vi "Capture ADC.vi"() -> ()   [LabVIEW 2023]
uses:
  <instrlib>/tio-labview/TIO Library/TIO Stream Open.vi
  <instrlib>/tio-labview/TIO Library/TIO RPC Send REQuest.vi
  <instrlib>/tio-labview/TIO Library/TIO RPC Parse Reply.vi
  <instrlib>/tio-labview/TIO Library/TIO RPC Parse Reply Error.vi
  <instrlib>/tio-labview/TIO Library/TIO Data Stream Parse timebase Info.vi
  <instrlib>/tio-labview/TIO Library/TIO Data Stream Parse pstream Info.vi
  <instrlib>/tio-labview/TIO Library/TIO Data Stream Parse dstream Info.vi
  <vilib>/Utility/High Resolution Relative Seconds.vi
  <vilib>/Utility/error.llb/Clear Errors.vi
  <instrlib>/tio-labview/Labview Signal Processing/Log Binning.vi
  <instrlib>/tio-labview/TIO Library/TIO Serial Port Name Search.vi
  <instrlib>/tio-labview/TIO Library/TIO Stream Write.vi
  <instrlib>/tio-labview/TIO Library/TIO RPC Form Request.vi
  <instrlib>/tio-labview/Labview Signal Processing/Log Range.vi
  <instrlib>/tio-labview/TIO Library/TIO SLIP Serial Write.vi
  <instrlib>/tio-labview/TIO Library/TIO Form Packet.vi
  <instrlib>/tio-labview/TIO Library/TIO SLIP Encode.vi
  <instrlib>/tio-labview/TIO Library/TIO Serial Checksum CRC32.vi
  <vilib>/Utility/tcp.llb/UDP Multicast Open.vi
  <vilib>/Utility/tcp.llb/UDP Multicast Read-Write Open.vi
  <instrlib>/tio-labview/TIO Library/TIO Serial Port Discovery.vi
  <vilib>/Instr/_visa.llb/VISA Configure Serial Port (Instr).vi
  <instrlib>/tio-labview/TIO Library/TIO RPC Blocking.vi
  <instrlib>/tio-labview/TIO Library/TIO Stream Read Non-blocking.vi
  <instrlib>/tio-labview/TIO Library/TIO RPC Send Heartbeat.vi
  <vilib>/Analysis/6fits.llb/General Polynomial Fit.vi
  <vilib>/measure/maspectr.llb/FFT Power Spectrum and PSD.vi
  <vilib>/measure/maspectr.llb/FFT Power Spectrum and PSD for 1 Chan.vi
panel:
  in  "Samples":u32
  in  "Auto Trigger":bool
  in  "Trigger":bool
  in  "Quit":bool
  out "ID":string
  in  "URL":refnum<visa-resource-name>="tcp://localhost"
  out "Waveform Graph":cluster{dbl, dbl, dbl[][]}(graph)
  in  "Bin":bool=TRUE
  out "XY Graph":T1(graph)=[{"Frequencies Binned"=[0.14367816091954022, 0.28735632183908044, 0.43103448275862066, 0.5747126436781609, 0.7183908045977011, 0.8620689655172413, 1.0057471264367814, 1.1494252873563218, 1.293103448275862, 1.4367816091954024, 1.5804597701149428, 1.724137931034483, 1.8678160919540234, 2.0114942528735638, 2.155172413793104, 2.2988505747126444, 2.4425287356321848, 2.586206896551725, 2.7298850574712654, 2.8735632183908058, 3.017241379310346, 3.1609195402298864, 3.3045977011494267, 3.448275862068967, 3.5919540229885074, 3.7356321839080477, 3.879310344827588, 4.022988505747128, 4.166666666666669, 4.310344827586209, 4.454022988505749, 4.59770114942529, 4.8132183908046, 5.028735632183911, 5.172413793103451, 5.316091954022991, 5.531609195402302, 5.747126436781612, 5.962643678160923, 6.178160919540233, 6.393678160919544, 6.6810344827586245, 6.896551724137935, 7.1120689655172455, 7.399425287356326, 7.686781609195407, 7.9741379310344875, 8.261494252873568, 8.548850574712649, 8.908045977011499, 9.267241379310349, 9.55459770114943, 9.91379310344828, 10.344827586206902, 10.704022988505752, 11.063218390804602, 11.494252873563227, 11.925287356321846, 12.356321839080467, 12.787356321839086, 13.290229885057478, 13.793103448275872, 14.295977011494262, 14.870689655172423, 15.445402298850585, 16.020114942528743, 16.5948275862069, 17.169540229885055, 17.816091954022976, 18.462643678160898, 19.10919540229882, 19.827586206896516, 20.54597701149421, 21.336206896551673, 22.126436781609133, 22.916666666666597, 23.778735632183825, 24.64080459770106, 25.57471264367806, 26.580459770114828, 27.586206896551598, 28.591954022988368, 29.597701149425138, 30.67528735632168, 31.824712643677987, 33.045977011494095, 34.26724137931019, 35.488505747126304, 36.85344827586195, 38.2183908045976, 39.58333333333324, 41.091954022988446, 42.600574712643635, 44.1810344827586, 45.83333333333334, 47.48563218390807, 49.28160919540235, 51.14942528735639, 53.017241379310434, 54.956896551724256, 56.96839080459785, 59.051724137931224, 61.27873563218412, 63.5775862068968, 65.94827586206915, 68.39080459770125, 70.9051724137931, 73.56321839080448, 76.29310344827564, 79.09482758620658, 82.04022988505704, 85.05747126436728, 88.14655172413728, 91.45114942528659, 94.89942528735543, 98.34770114942428, 101.93965517241267, 105.74712643678036, 109.69827586206759, 113.79310344827434, 117.95977011494085, 122.27011494252692, 126.86781609195204, 131.6091954022967, 136.42241379310113, 141.45114942528483, 146.69540229884782, 152.15517241379015, 157.8304597701118, 163.64942528735295, 169.6839080459734, 176.00574712643294, 182.5431034482718, 189.29597701148995, 196.2643678160874], "Spectrum Binned"=[nan, nan, nan, nan, nan, nan, nan, nan, nan, nan, nan, nan, nan, nan, nan, nan, nan, nan, nan, nan, nan, nan, nan, nan, nan, nan, nan, nan, nan, nan, nan, nan, nan, nan, nan, nan, nan, nan, nan, nan, nan, nan, nan, nan, nan, nan, nan, nan, nan, nan, nan, nan, nan, nan, nan, nan, nan, nan, nan, nan, nan, nan, nan, nan, nan, nan, nan, nan, nan, nan, nan, nan, nan, nan, nan, nan, nan, nan, nan, nan, nan, nan, nan, nan, nan, nan, nan, nan, nan, nan, nan, nan, nan, nan, nan, nan, nan, nan, nan, nan, nan, nan, nan, nan, nan, nan, nan, nan, nan, nan, nan, nan, nan, nan, nan, nan, nan, nan, nan, nan, nan, nan, nan, nan, nan, nan, nan, nan, nan, nan, nan, nan, nan, nan, nan]}, {"Frequencies Binned"=[0.14367816091954022, 0.28735632183908044, 0.43103448275862066, 0.5747126436781609, 0.7183908045977011, 0.8620689655172413, 1.0057471264367814, 1.1494252873563218, 1.293103448275862, 1.4367816091954024, 1.5804597701149428, 1.724137931034483, 1.8678160919540234, 2.0114942528735638, 2.155172413793104, 2.2988505747126444, 2.4425287356321848, 2.586206896551725, 2.7298850574712654, 2.8735632183908058, 3.017241379310346, 3.1609195402298864, 3.3045977011494267, 3.448275862068967, 3.5919540229885074, 3.7356321839080477, 3.879310344827588, 4.022988505747128, 4.166666666666669, 4.310344827586209, 4.454022988505749, 4.59770114942529, 4.8132183908046, 5.028735632183911, 5.172413793103451, 5.316091954022991, 5.531609195402302, 5.747126436781612, 5.962643678160923, 6.178160919540233, 6.393678160919544, 6.6810344827586245, 6.896551724137935, 7.1120689655172455, 7.399425287356326, 7.686781609195407, 7.9741379310344875, 8.261494252873568, 8.548850574712649, 8.908045977011499, 9.267241379310349, 9.55459770114943, 9.91379310344828, 10.344827586206902, 10.704022988505752, 11.063218390804602, 11.494252873563227, 11.925287356321846, 12.356321839080467, 12.787356321839086, 13.290229885057478, 13.793103448275872, 14.295977011494262, 14.870689655172423, 15.445402298850585, 16.020114942528743, 16.5948275862069, 17.169540229885055, 17.816091954022976, 18.462643678160898, 19.10919540229882, 19.827586206896516, 20.54597701149421, 21.336206896551673, 22.126436781609133, 22.916666666666597, 23.778735632183825, 24.64080459770106, 25.57471264367806, 26.580459770114828, 27.586206896551598, 28.591954022988368, 29.597701149425138, 30.67528735632168, 31.824712643677987, 33.045977011494095, 34.26724137931019, 35.488505747126304, 36.85344827586195, 38.2183908045976, 39.58333333333324, 41.091954022988446, 42.600574712643635, 44.1810344827586, 45.83333333333334, 47.48563218390807, 49.28160919540235, 51.14942528735639, 53.017241379310434, 54.956896551724256, 56.96839080459785, 59.051724137931224, 61.27873563218412, 63.5775862068968, 65.94827586206915, 68.39080459770125, 70.9051724137931, 73.56321839080448, 76.29310344827564, 79.09482758620658, 82.04022988505704, 85.05747126436728, 88.14655172413728, 91.45114942528659, 94.89942528735543, 98.34770114942428, 101.93965517241267, 105.74712643678036, 109.69827586206759, 113.79310344827434, 117.95977011494085, 122.27011494252692, 126.86781609195204, 131.6091954022967, 136.42241379310113, 141.45114942528483, 146.69540229884782, 152.15517241379015, 157.8304597701118, 163.64942528735295, 169.6839080459734, 176.00574712643294, 182.5431034482718, 189.29597701148995, 196.2643678160874], "Spectrum Binned"=[nan, nan, nan, nan, nan, nan, nan, nan, nan, nan, nan, nan, nan, nan, nan, nan, nan, nan, nan, nan, nan, nan, nan, nan, nan, nan, nan, nan, nan, nan, nan, nan, nan, nan, nan, nan, nan, nan, nan, nan, nan, nan, nan, nan, nan, nan, nan, nan, nan, nan, nan, nan, nan, nan, nan, nan, nan, nan, nan, nan, nan, nan, nan, nan, nan, nan, nan, nan, nan, nan, nan, nan, nan, nan, nan, nan, nan, nan, nan, nan, nan, nan, nan, nan, nan, nan, nan, nan, nan, nan, nan, nan, nan, nan, nan, nan, nan, nan, nan, nan, nan, nan, nan, nan, nan, nan, nan, nan, nan, nan, nan, nan, nan, nan, nan, nan, nan, nan, nan, nan, nan, nan, nan, nan, nan, nan, nan, nan, nan, nan, nan, nan, nan, nan, nan]}, {"Frequencies Binned"=[0.14367816091954022, 0.28735632183908044, 0.43103448275862066, 0.5747126436781609, 0.7183908045977011, 0.8620689655172413, 1.0057471264367814, 1.1494252873563218, 1.293103448275862, 1.4367816091954024, 1.5804597701149428, 1.724137931034483, 1.8678160919540234, 2.0114942528735638, 2.155172413793104, 2.2988505747126444, 2.4425287356321848, 2.586206896551725, 2.7298850574712654, 2.8735632183908058, 3.017241379310346, 3.1609195402298864, 3.3045977011494267, 3.448275862068967, 3.5919540229885074, 3.7356321839080477, 3.879310344827588, 4.022988505747128, 4.166666666666669, 4.310344827586209, 4.454022988505749, 4.59770114942529, 4.8132183908046, 5.028735632183911, 5.172413793103451, 5.316091954022991, 5.531609195402302, 5.747126436781612, 5.962643678160923, 6.178160919540233, 6.393678160919544, 6.6810344827586245, 6.896551724137935, 7.1120689655172455, 7.399425287356326, 7.686781609195407, 7.9741379310344875, 8.261494252873568, 8.548850574712649, 8.908045977011499, 9.267241379310349, 9.55459770114943, 9.91379310344828, 10.344827586206902, 10.704022988505752, 11.063218390804602, 11.494252873563227, 11.925287356321846, 12.356321839080467, 12.787356321839086, 13.290229885057478, 13.793103448275872, 14.295977011494262, 14.870689655172423, 15.445402298850585, 16.020114942528743, 16.5948275862069, 17.169540229885055, 17.816091954022976, 18.462643678160898, 19.10919540229882, 19.827586206896516, 20.54597701149421, 21.336206896551673, 22.126436781609133, 22.916666666666597, 23.778735632183825, 24.64080459770106, 25.57471264367806, 26.580459770114828, 27.586206896551598, 28.591954022988368, 29.597701149425138, 30.67528735632168, 31.824712643677987, 33.045977011494095, 34.26724137931019, 35.488505747126304, 36.85344827586195, 38.2183908045976, 39.58333333333324, 41.091954022988446, 42.600574712643635, 44.1810344827586, 45.83333333333334, 47.48563218390807, 49.28160919540235, 51.14942528735639, 53.017241379310434, 54.956896551724256, 56.96839080459785, 59.051724137931224, 61.27873563218412, 63.5775862068968, 65.94827586206915, 68.39080459770125, 70.9051724137931, 73.56321839080448, 76.29310344827564, 79.09482758620658, 82.04022988505704, 85.05747126436728, 88.14655172413728, 91.45114942528659, 94.89942528735543, 98.34770114942428, 101.93965517241267, 105.74712643678036, 109.69827586206759, 113.79310344827434, 117.95977011494085, 122.27011494252692, 126.86781609195204, 131.6091954022967, 136.42241379310113, 141.45114942528483, 146.69540229884782, 152.15517241379015, 157.8304597701118, 163.64942528735295, 169.6839080459734, 176.00574712643294, 182.5431034482718, 189.29597701148995, 196.2643678160874], "Spectrum Binned"=[nan, nan, nan, nan, nan, nan, nan, nan, nan, nan, nan, nan, nan, nan, nan, nan, nan, nan, nan, nan, nan, nan, nan, nan, nan, nan, nan, nan, nan, nan, nan, nan, nan, nan, nan, nan, nan, nan, nan, nan, nan, nan, nan, nan, nan, nan, nan, nan, nan, nan, nan, nan, nan, nan, nan, nan, nan, nan, nan, nan, nan, nan, nan, nan, nan, nan, nan, nan, nan, nan, nan, nan, nan, nan, nan, nan, nan, nan, nan, nan, nan, nan, nan, nan, nan, nan, nan, nan, nan, nan, nan, nan, nan, nan, nan, nan, nan, nan, nan, nan, nan, nan, nan, nan, nan, nan, nan, nan, nan, nan, nan, nan, nan, nan, nan, nan, nan, nan, nan, nan, nan, nan, nan, nan, nan, nan, nan, nan, nan, nan, nan, nan, nan, nan, nan]}]
  # "Capture"
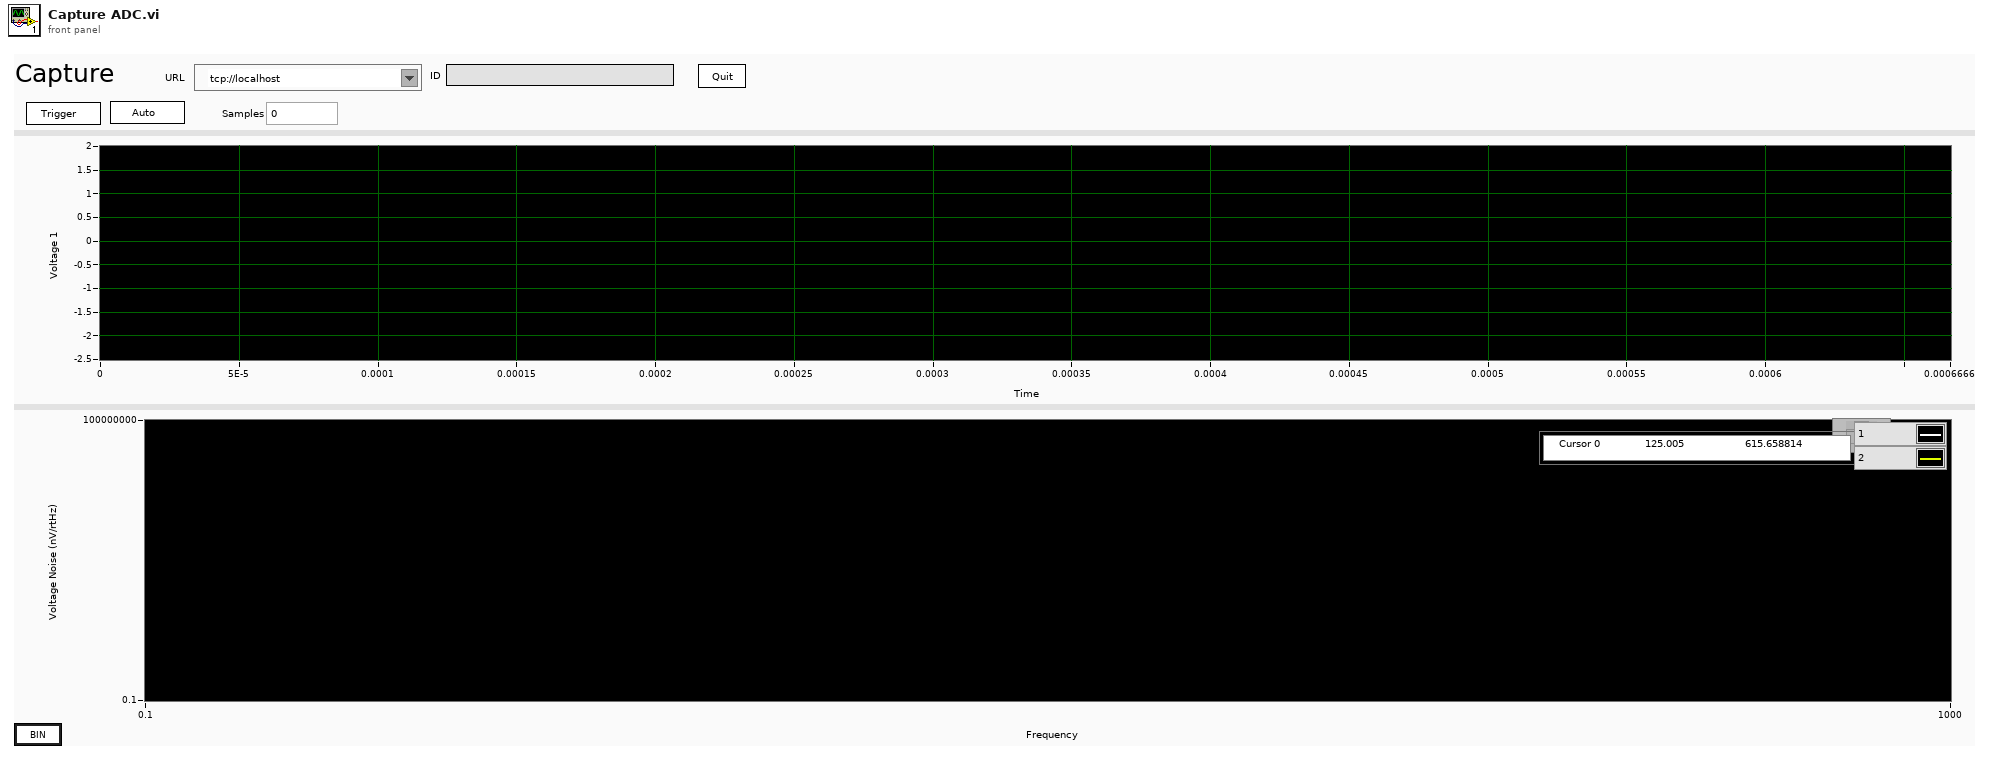
[diagram p1: front panel]
types:
  T1 = cluster{"Frequencies Binned":dbl[], "Spectrum Binned":dbl[]}[]
  T2 = cluster{"TS Connection":cluster{"Type":enum16{"Serial", "TCP", "UDP", "mUDP"}, "URL":refnum<visa-resource-name>, "TO":u32, "Addr":u32, "Port":i32, "TCP":refnum<k5>, "UDP":refnum<k16>, "Route":string}, "REQ":refnum<queue>, "REP":refnum<queue>}
  T3 = enum16{"big-endian, network order", "native, host order", "little-endian"}
  T4 = cluster{"Awaiting REP":bool, "REQ ID":u32, "streams in":cluster{"id":u16, "timebase id":u16, "period":u32, "offset":u32, "sample number":u64, "total components":u16, "flags":u16, "components":cluster{"source id":u16, "flags":u16, "period":u32, "offset":u32}[]}[], "sources":cluster{"id":u16, "timebase_id":u16, "period":u32, "offset":u32, "fmt":i32, "flags":u16, "channels":u16, "type":u8, "name":string, "column names":string[], "title":string, "units":string}[], "timebases":cluster{"id":u16, "source":u8, "epoch":u8, "start time":u64, "period numerator (µs)":u32, "period denominator (µs)":u32, "flags":u32, "stability":sgl, "source id":string}[]}
  T5 = cluster{"TC Connection":cluster{"Type":enum16{"Serial", "TCP", "UDP", "mUDP"}, "URL":refnum<visa-resource-name>, "TO":u32, "Addr":u32, "Port":i32, "TCP":refnum<k5>, "UDP":refnum<k16>, "Route":string}, "REQ":refnum<queue>, "REP":refnum<queue>}
  T6 = cluster{"Frequencies Binned":dbl[], "Spectrum Binned":dbl[]}
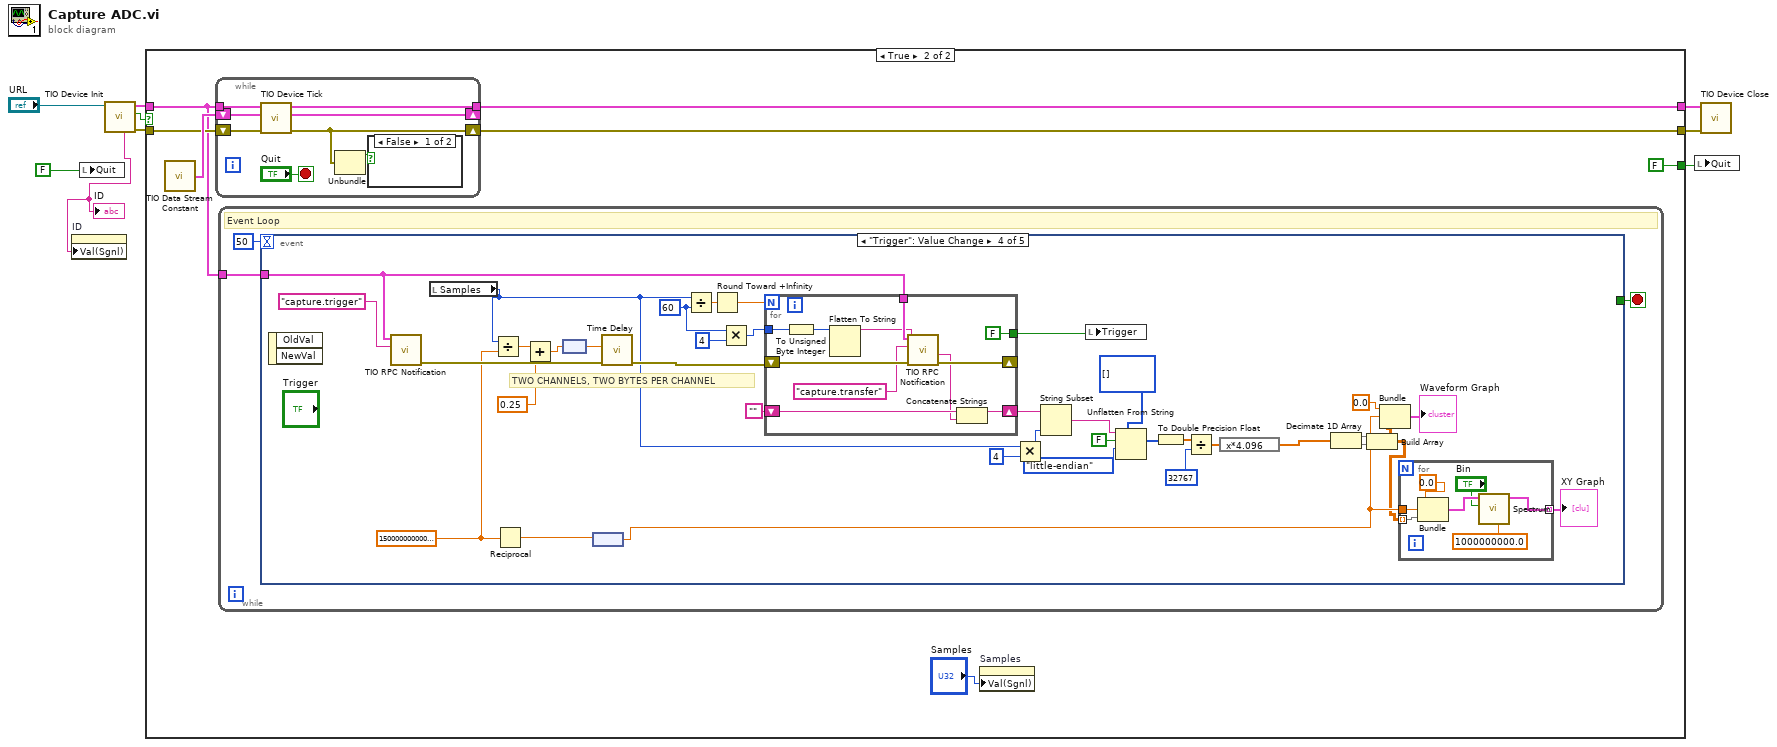
[diagram p0: block diagram]
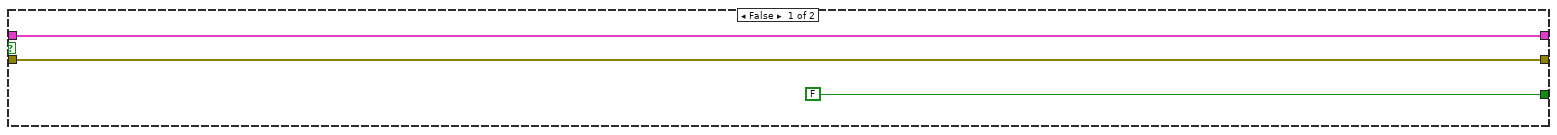
[diagram p2: hidden frame]
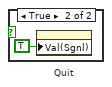
[diagram p3: hidden frame]
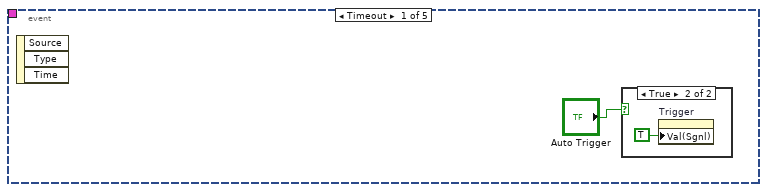
[diagram p4: hidden frame]
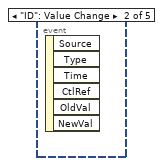
[diagram p6: hidden frame]
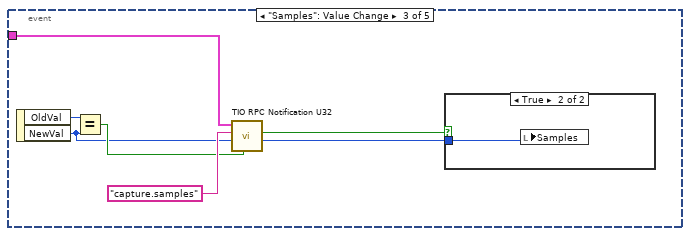
[diagram p7: hidden frame]
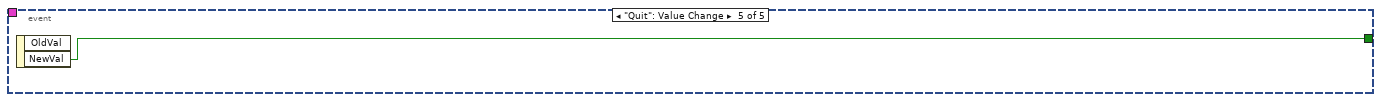
[diagram p9: hidden frame]
diagram:
  n1 = local write "Quit"(FALSE ("Quit")) -> ()
  n2 = call <instrlib>:"TIO Device Init.vi"("URL"="URL") -> ("error out"=w6:errorcluster, 2:"ID Verified"=w7:bool, "TIO"=w8:T2, 4:"ID Verified"=w2:string)  [unwired: 6 in, 1 out]
  "ID" <- w2
  n3 = property on="ID" class="Str"("Val(Sgnl)"=w2) -> ()  [unwired: 2 in, 2 out]
  n4 = case shown="True" w7 {
    tunnel: w8 -> [w12 w13]
    tunnel: w6 -> [w11 w14]
    tunnel: [w11 w19] -> w4
    tunnel: [w12 w18] -> w3
    tunnel: [FALSE ("Quit") FALSE ("Quit")] -> w1
    frame False {
    }
    frame True {
      n5 = call <instrlib>:"TIO Data Stream Constant.vi"() -> ("TIO State"=w16:T4)
      n6 = while {
        tunnel: w13 -> [w26]
        shift-right: [w24] -> _
        shift-left: w16 -> [w23]
        tunnel: [w22] -> w18
        shift-right: [w21] -> w19
        shift-left: w14 -> [w27]
        stop <- "Quit" stop-if-true
        n7 = call <instrlib>:"TIO Device Tick.vi"("Error in"=w27, "TIO State"=w23, "TIO"=w26) -> ("Error out"=w21:errorcluster, "TIO State"=w24:T4, "TIO"=w22:T5)  [unwired: 5 in, 1 out]
        n8 = Unbundle(w21) -> ("status"=w20:bool)  [unwired: 2 out]
        n9 = case shown="False" w20 {
          frame False {
          }
          frame True {
            n10 = property on="Quit" class="Bool (strict)"("Val(Sgnl)"=TRUE ("Value (Signaling)")) -> ()  [unwired: 2 in, 2 out]
          }
        }
      }
      n11 = while {
        tunnel: w13 -> [w30]
        stop <- w29 stop-if-true
        # "Event Loop"
        n12 = event shown="[3] \"Trigger\": Value Change" {
          selector: _ -> [_ _ _ _ _]
          dyn-events: _ -> [_ _ _ _ _]
          timeout: 50 -> [_ _ _ _ _]
          tunnel: w30 -> [_ _ w39 w71 _]
          tunnel: [_ _ _ _ w97] -> w29
          event Timeout {
            n13 = event-data() -> ()  [unwired: 1 in, 3 out]
            n14 = case shown="True" "Auto Trigger" {
              frame False {
              }
              frame True {
                n15 = property on="Trigger" class="Bool (strict)"("Val(Sgnl)"=TRUE ("Value (Signaling)")) -> ()  [unwired: 2 in, 2 out]
              }
            }
          }
          event "ID": Value Change {
            n16 = event-data() -> ()  [unwired: 1 in, 6 out]
          }
          event "Samples": Value Change {
            n17 = event-data() -> ("OldVal"=w38:u32, "NewVal"=w36:u32)  [unwired: 1 in]
            n18 = Equal?(x=w38, y=w36) -> (x = y?=w37:bool)
            n19 = call <instrlib>:"TIO RPC Notification U32.vi"("Read"=w37, "Set value"=w36, "Topic"="capture.samples", "TIO"=w39) -> ("Get value (default if error)"=w34:u32, "Response"=w35:bool)  [unwired: 4 in, 1 out]
            n20 = case shown="True" w35 {
              tunnel: w34 -> [_ w41]
              frame False {
              }
              frame True {
                n21 = local write "Samples"(w41) -> ()
              }
            }
          }
          event "Trigger": Value Change {
            w62 = u32 60 ("Samples")
            w69 = dbl[unit] 15000000000000.0 ("Delay Time (s)")
            # "TWO CHANNELS, TWO BYTES PER CHANNEL"
            n22 = event-data() -> ()  [unwired: 1 in, 2 out]
            n23 = call <instrlib>:"TIO RPC Notification.vi"("Topic"="capture.trigger", "TIO"=w71) -> ("error out"=w72:errorcluster)  [unwired: 6 in, 2 out]
            n24 = local read "Samples"() -> (w55:u32)
            n25 = Divide(x=w55, y=w69) -> (x/y=w49:dbl[unit])
            n26 = Reciprocal(x=w69) -> (1/x=w68:dbl[unit])
            n27 = Add(x=w49, y=dbl[unit] 0.25) -> (x+y=w48:dbl[unit])
            n28 = node(w48) -> (w70:dbl)
            n29 = node(w68) -> (w51:dbl)
            n30 = call "Time Delay"("error in (no error)"=w72, "Delay Time (s)"=w70) -> ("error out"=w65:errorcluster)  [unwired: 9 in]
            n31 = Divide(x=w55, y=w62) -> (x/y=w77:dbl)
            n32 = Round Toward +Infinity(x=w77) -> (ceil(x): smallest int >= x=w64:dbl)
            n33 = Multiply(x=w62, y=u32 4) -> (x*y=w61:u32)
            n34 = for {
              N: w64 -> [_]
              shift-right: [w96] -> _
              shift-left: w65 -> [w95]
              tunnel: w71 -> [w93]
              shift-right: [w92] -> w59
              shift-left: "" -> [w91]
              tunnel: [FALSE ("Trigger")] -> w76
              tunnel: w61 -> [w87]
              n35 = To Unsigned Byte Integer(number=w87) -> (unsigned 8bit integer=w88:u8)
              n36 = Flatten To String(anything=w88) -> (data string=w86:string)  [unwired: 3 in, 2 out]
              n37 = call <instrlib>:"TIO RPC Notification.vi"("error in (no error)"=w95, "Payload"=w86, "Topic"="capture.transfer", "TIO"=w93) -> ("error out"=w96:errorcluster, "REP"=w90:string)  [unwired: 4 in, 1 out]
              n38 = Concatenate Strings(w91, w90) -> (w92:string)
            }
            n39 = Multiply(x=w55, y=u32 4) -> (x*y=w56:u32)
            n40 = String Subset(string=w59, length (rest)=w56) -> (substring=w58:string)  [unwired: 1 in]
            n41 = local write "Trigger"(w76) -> ()
            n42 = Unflatten From String(type=i16[] [], binary string=w58, data includes array or string size? (T)=FALSE, byte order (0:big-endian, network order)=T3."little-endian") -> (value=w46:i16[])  [unwired: 1 in, 2 out]
            n43 = To Double Precision Float(number=w46) -> (double precision float=w45:dbl[])
            n44 = Divide(x=w45, y=u16 32767) -> (x/y=w43:dbl[])
            n45 = expression code="x*4.096"(w43) -> (w42:dbl[])
            n46 = Decimate 1D Array(w42) -> (w54:dbl[], w53:dbl[])
            n47 = Build Array(w54, w53) -> (w50:dbl[][])
            n48 = Bundle(0.0, w51, w50) -> (→"Waveform Graph":cluster{dbl, dbl, dbl[][]})  [unwired: 1 in]
            n49 = for {
              tunnel: [w85] -> w52 mode=indexing
              tunnel: w51 -> [w82]
              tunnel: w50 -> [w81] mode=indexing
              n50 = Bundle(0.0, w82, w81) -> (w84:cluster{dbl, dbl, dbl[]})  [unwired: 1 in]
              n51 = call <instrlib>:"Spectrum.vi"("Gain"=1000000000.0, "Binning"="Bin", "Waveform 1"=w84) -> ("Cluster"=w85:T6)  [unwired: 6 in]
            }
            "XY Graph" <- w52
          }
          event "Quit": Value Change {
            n52 = event-data() -> ("NewVal"=w97:bool)  [unwired: 1 in, 1 out]
          }
        }
      }
      n53 = property on="Samples" class="DigNum (strict)"("Val(Sgnl)"="Samples") -> ()  [unwired: 2 in, 2 out]
    }
  }
  n54 = local write "Quit"(w1) -> ()
  n55 = call <instrlib>:"TIO Device Close.vi"("Error in"=w4, "TIO"=w3) -> ()  [unwired: 10 in]
